vi "Local Trajectory Loading.vi"(6 "PID Cluster":T4={"L1 to L4 PID Cluster"={"L1 PID Gains"={"Kp"=0.005, "Kd"=0.5, "Ki"=0.0005}, "L2 PID Gains"={"Kp"=0.01, "Kd"=1.0, "Ki"=0.005}, "L3 PID Gains"={"Kp"=0.05, "Kd"=1.0, "Ki"=0.0005}, "L4 PID Gains"={"Kp"=0.1, "Kd"=0.1, "Ki"=0.0005}}, "Stage PID Cluster"={"Stage Z PID"={"Kp"=0.0005, "Kd"=0.001, "Ki"=0.0}, "Stage Y PID"={"Kp"=0.0003, "Kd"=0.01, "Ki"=0.0}, "Stage X PID"={"Kp"=0.0003, "Kd"=0.01, "Ki"=0.0}}, "OCT Z PID Gains"={"Kp"=0.0003, "Kd"=0.0001, "Ki"=0.01}}, 8 "error in":errorcluster, 9 "Offset Home 2 RCM":dbl[](array[numeric])=[0.0, 0.0, 0.0, 0.0], 10 "Prev Posit Cluster":T3={"Prev L1 to L4 Posit"=[-0.5319, -0.035669172703475985, -2.0566170657346783, 0.9099264705882353], "Prev Stage Posit"=[6.002553885707208, 5.996566124542428, 5.995469940427586], "Prev OCT Z Posit"=-0.0}, 11 "FPGA VI Reference In":refnum<k20>) -> (1 "Trajectory Cluster":T1, 2 "Last Posit Cluster":T2={"Last L1 to L4 Posit"=[0.0, 0.0, 0.0, 0.0], "Last Stage Posit"=[6.0, 6.0, 6.0], "Last OCT Z Posit"=0.0}, 3 "FPGA VI Reference Out":refnum<k20>, 4 "error out":errorcluster, 5 "First Trk Pt":dbl[](array[numeric]))   [LabVIEW 2016]
uses:
  <vilib>/Platform/TimedLoop/XDataNode/timing_clust.ctl
  <vilib>/Platform/TimedLoop/XDataNode/nitl_modes.ctl
  <vilib>/Platform/TimedLoop/XDataNode/wakeup.ctl
  Global Variables.vi
  <vilib>/platform/TimedLoop/XDataNode/XDataNode.xnode
  <vilib>/Platform/TimedLoop/XDataNode/XDNodeRunTimeDep.lvlib
panel:
  out "In Servo Loop":bool
  out "Loading Finished":bool
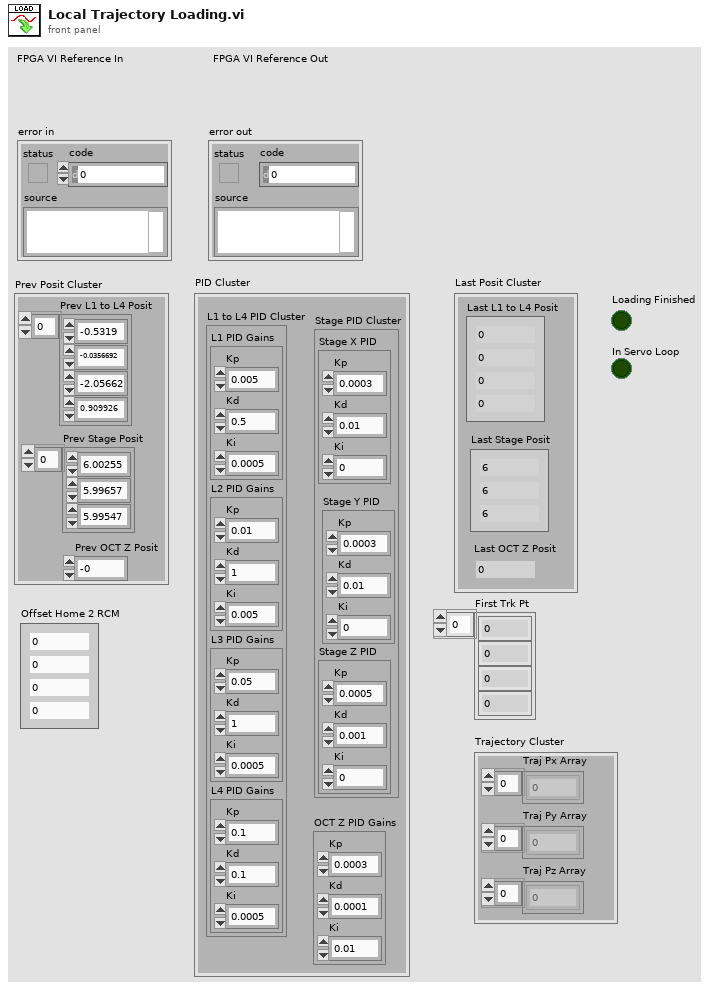
[diagram p1: front panel]
types:
  T1 = cluster{"Traj Px Array":dbl[], "Traj Py Array":dbl[], "Traj Pz Array":dbl[]}
  T2 = cluster{"Last L1 to L4 Posit":dbl[], "Last Stage Posit":dbl[], "Last OCT Z Posit":dbl}
  T3 = cluster{"Prev L1 to L4 Posit":dbl[], "Prev Stage Posit":dbl[], "Prev OCT Z Posit":dbl}
  T4 = cluster{"L1 to L4 PID Cluster":cluster{"L1 PID Gains":cluster{"Kp":dbl, "Kd":dbl, "Ki":dbl}, "L2 PID Gains":cluster{"Kp":dbl, "Kd":dbl, "Ki":dbl}, "L3 PID Gains":cluster{"Kp":dbl, "Kd":dbl, "Ki":dbl}, "L4 PID Gains":cluster{"Kp":dbl, "Kd":dbl, "Ki":dbl}}, "Stage PID Cluster":cluster{"Stage Z PID":cluster{"Kp":dbl, "Kd":dbl, "Ki":dbl}, "Stage Y PID":cluster{"Kp":dbl, "Kd":dbl, "Ki":dbl}, "Stage X PID":cluster{"Kp":dbl, "Kd":dbl, "Ki":dbl}}, "OCT Z PID Gains":cluster{"Kp":dbl, "Kd":dbl, "Ki":dbl}}
  T5 = typedef "XDNodeRunTimeDep.lvlib/timing_clust.ctl" = cluster{"Expected End [f-1]":u64, "Actual End [f-1]":u64, "Finished Late? [f-1]":bool, "Expected End [i-1]":u64, "Actual End [i-1]":u64, "Finished Late? [i-1]":bool, "Expected Start [i]":u64, "Actual Start [i]":u64, "Expected Start [f]":u64, "Actual Start [f]":u64, "Source Name":string, "Structure Name":string, "Period":i64, "Deadline":i64, "Offset":i64, "Start":i64, "Priority":i32, "Timeout":i32, "Mode":T6, "Wakeup Reason":T7, "Error":errorcluster, "Source Type":string, "Secondary Source Type":string, "Global End Time":u64, "Global Start Time":u64, "Frame Duration":u64, "Iteration Duration":u64, "Assigned CPU":i32, "I/O Scan Engine Mode":u32}
  T6 = typedef "XDNodeRunTimeDep.lvlib/nitl_modes.ctl" = enum32{"No Change", "Process missed periods, maintain original phase", "Discard missed periods, maintain original phase", "Process missed periods, ignore original phase", "Discard missed periods, ignore original phase"}
  T7 = typedef "XDNodeRunTimeDep.lvlib/wakeup.ctl" = enum32{"Normal", "Aborted", "Asynchronous wakeup", "Timing source error", "Timed loop error", "Timeout"}
  T8 = cluster{"L1 PID Gains":cluster{"Kp":dbl, "Kd":dbl, "Ki":dbl}, "L2 PID Gains":cluster{"Kp":dbl, "Kd":dbl, "Ki":dbl}, "L3 PID Gains":cluster{"Kp":dbl, "Kd":dbl, "Ki":dbl}, "L4 PID Gains":cluster{"Kp":dbl, "Kd":dbl, "Ki":dbl}}
  T9 = cluster{"Stage Z PID":cluster{"Kp":dbl, "Kd":dbl, "Ki":dbl}, "Stage Y PID":cluster{"Kp":dbl, "Kd":dbl, "Ki":dbl}, "Stage X PID":cluster{"Kp":dbl, "Kd":dbl, "Ki":dbl}}
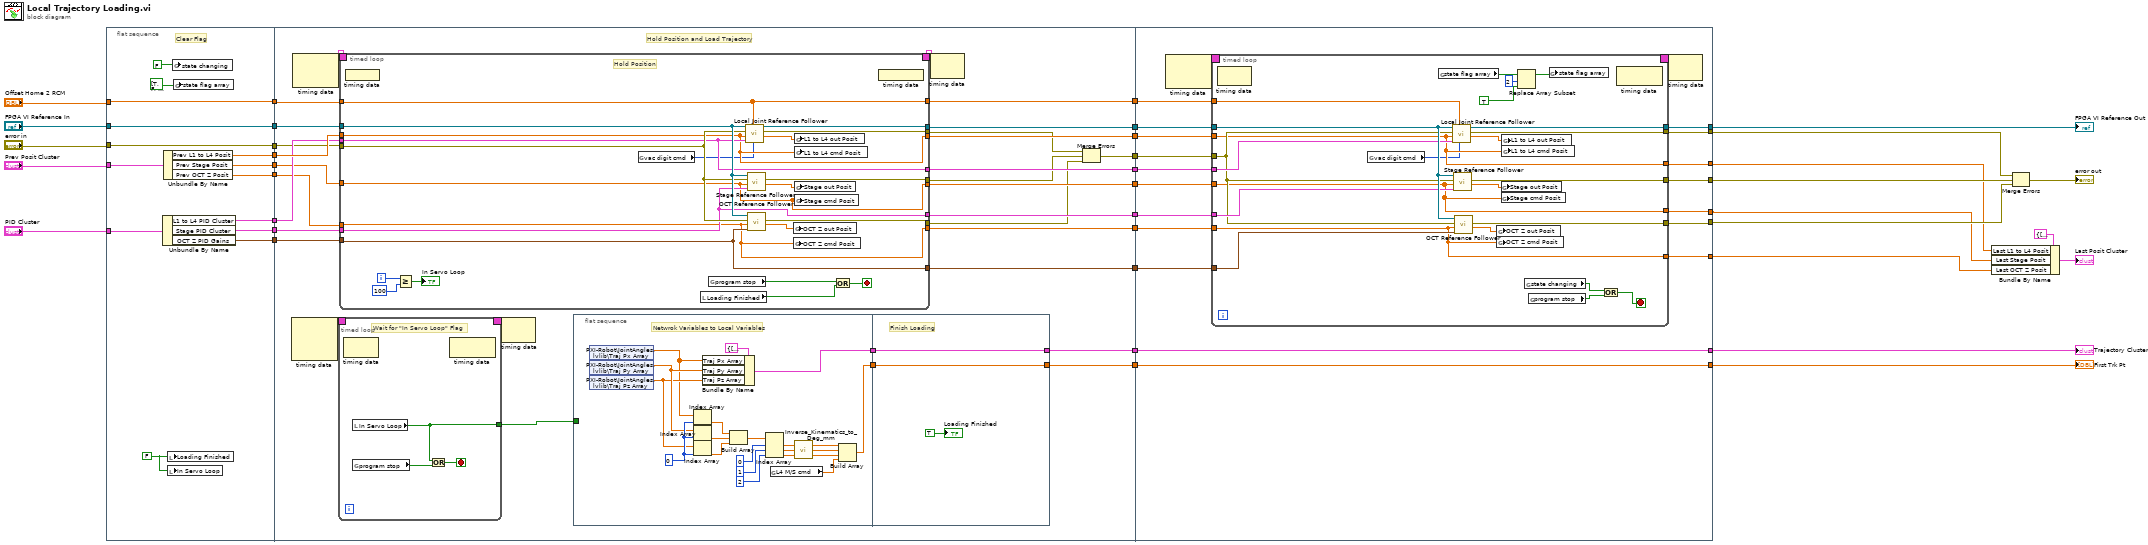
[diagram p0: block diagram]
diagram:
  n1 = flat-sequence {
    tunnel: [w49] -> w37
    tunnel: "FPGA VI Reference In" -> [w49]
    tunnel: [w48] -> w35
    tunnel: "error in" -> [w48]
    tunnel: "Prev Posit Cluster" -> [w47]
    tunnel: "PID Cluster" -> [w46]
    tunnel: [w45] -> w33
    tunnel: [w44] -> w32
    tunnel: "Offset Home 2 RCM" -> [w43]
    tunnel: [w43] -> w30
    tunnel: [w42] -> w27
    tunnel: [w41] -> w26
    tunnel: [w40] -> w25
    tunnel: [w39] -> w24
    tunnel: w37 -> [w67]
    tunnel: w35 -> [w62]
    tunnel: w33 -> [w64]
    tunnel: w32 -> [w63]
    tunnel: w30 -> [w68]
    tunnel: w27 -> [w66]
    tunnel: w26 -> [w61]
    tunnel: w25 -> [w60]
    tunnel: w24 -> [w65]
    tunnel: [w81] -> w12
    tunnel: [w80] -> w11
    tunnel: [w79] -> w10
    tunnel: [w78] -> w9
    tunnel: [w77] -> w8
    tunnel: [w76] -> w7
    tunnel: [w75] -> w6
    tunnel: [w74] -> w5
    tunnel: [w56] -> w4
    tunnel: [w55] -> w3
    tunnel: [w54] -> w2
    tunnel: w12 -> [w157]
    tunnel: [w156] -> w22
    tunnel: [w155] -> w21
    tunnel: [w154] -> w20
    tunnel: w11 -> [w153]
    tunnel: w10 -> [w152]
    tunnel: w9 -> [w151]
    tunnel: w8 -> [w150]
    tunnel: w7 -> [w149]
    tunnel: w6 -> [w148]
    tunnel: w5 -> [w147]
    tunnel: [w146] -> w18
    tunnel: [w145] -> w17
    tunnel: [w144] -> w16
    tunnel: [w143] -> w14
    tunnel: [w140] -> w13
    tunnel: w4 -> [w142]
    tunnel: w3 -> [w140]
    tunnel: [w141] -> w1
    tunnel: w2 -> [w141]
    frame #0 {
      w38 = FALSE ("Loading Finished")
      # "Clear Flag"
      n2 = Unbundle By Name(w46) -> ("L1 to L4 PID Cluster"=w44:T8, "Stage PID Cluster"=w45:T9, "OCT Z PID Gains"=w39:cluster{"Kp":dbl, "Kd":dbl, "Ki":dbl})
      n3 = Unbundle By Name(w47) -> ("Prev L1 to L4 Posit"=w42:dbl[], "Prev Stage Posit"=w41:dbl[], "Prev OCT Z Posit"=w40:dbl)
      n4 = local write "Loading Finished"(w38) -> ()
      n5 = local write "In Servo Loop"(w38) -> ()
      n6 = global write "Global Variables.vi" "state changing"(FALSE ("state changing")) -> ()
      n7 = global write "Global Variables.vi" "state flag array"(bool[] [TRUE, FALSE, FALSE, FALSE, FALSE, FALSE, FALSE, FALSE, FALSE] ("state flag array")) -> ()
    }
    frame #1 {
      # "Hold Position and Load Trajectory"
      n8 = node-c288() -> (w71:T5)  [unwired: 3 in]
      n9 = node-c288() -> (w73:T5)  [unwired: 2 in]
      n10 = timed-loop {
        timing: w71 -> [_]
        timing-out: [_] -> w70
        tunnel: [w83] -> w69
        stop <- w84 stop-if-true
        # "Wait for \"In Servo Loop\" Flag"
        n11 = node-c288() -> ()  [unwired: 1 in, 1 out]
        n12 = local read "In Servo Loop"() -> (w83:bool)
        n13 = global read "Global Variables.vi" "program stop"() -> (w82:bool)
        n14 = Or(x=w83, y=w82) -> (x .or. y?=w84:bool)
        n15 = node-c288() -> ()  [unwired: 1 in, 1 out]
      }
      n16 = timed-loop {
        timing: w73 -> [_]
        timing-out: [_] -> w72
        tunnel: w66 -> [w116]
        tunnel: w61 -> [w115]
        tunnel: w64 -> [w120]
        tunnel: w63 -> [w121]
        tunnel: w62 -> [w131]
        tunnel: w67 -> [w132]
        tunnel: w68 -> [w127]
        tunnel: w60 -> [w114]
        tunnel: w65 -> [w122]
        tunnel: [w116] -> w79
        tunnel: [w115] -> w78
        tunnel: [w114] -> w77
        tunnel: [w127] -> w80
        tunnel: [w126] -> w81
        tunnel: [w125] -> w59
        tunnel: [w124] -> w58
        tunnel: [w123] -> w57
        tunnel: [w122] -> w76
        tunnel: [w121] -> w75
        tunnel: [w120] -> w74
        i -> [w119]
        stop <- w135 stop-if-true
        # "Hold Position"
        n17 = node-c288 ("Output Node")() -> ()  [unwired: 1 in]
        n18 = Greater Or Equal?(x=w119, y=100) -> (x >= y?=→"In Servo Loop":bool)
        n19 = global read "Global Variables.vi" "vac digit cmd"() -> (w113:i8)
        n20 = local read "Loading Finished"() -> (w134:bool)
        n21 = global read "Global Variables.vi" "program stop"() -> (w133:bool)
        n22 = call "Local Joint Reference Follower.vi"("Digital Cmd [0-78]"=w113, "Offset Home2RCM [deg/mm]"=w127, "PID Ctrl Cluster"=w121, "Ref Array [deg/mm]"=w116, "error in"=w131, "FPGA VI Reference In"=w132) -> ("Output Posit Array [deg/mm]"=w130:dbl[], "error out"=w125:errorcluster, "FPGA VI Reference Out"=w126:refnum<k20>)  [unwired: 3 in]
        n23 = call "Stage Reference Follower.vi"("Stage PID Cluster"=w120, "Stage cmd Posit [mm]"=w115, "error in"=w131, "FPGA VI Reference In"=w132) -> ("Stage out Posit [mm]"=w129:dbl[], "error out"=w124:errorcluster)  [unwired: 5 in, 1 out]
        n24 = call "OCT Reference Follower.vi"("OCT Z PID Gains"=w122, "OCT  Z cmd Posit [mm]"=w114, "error in"=w131, "FPGA VI Reference In"=w132) -> ("OCT  Z out Posit [mm]"=w128:dbl, "error out"=w123:errorcluster)  [unwired: 5 in, 1 out]
        n25 = global write "Global Variables.vi" "OCT Z out Posit"(w128) -> ()
        n26 = global write "Global Variables.vi" "OCT Z cmd Posit"(w114) -> ()
        n27 = global write "Global Variables.vi" "L1 to L4 out Posit"(w130) -> ()
        n28 = global write "Global Variables.vi" "L1 to L4 cmd Posit"(w116) -> ()
        n29 = global write "Global Variables.vi" "Stage out Posit"(w129) -> ()
        n30 = global write "Global Variables.vi" "Stage cmd Posit"(w115) -> ()
        n31 = Or(x=w133, y=w134) -> (x .or. y?=w135:bool)
        n32 = node-c288() -> ()  [unwired: 1 out]
      }
      n33 = node-c288(w70) -> ()  [unwired: 1 out]
      n34 = flat-sequence {
        tunnel: [w108] -> w53
        tunnel: w69 -> [_]
        tunnel: [w91] -> w52
        tunnel: w53 -> [w111]
        tunnel: [w111] -> w55
        tunnel: [w110] -> w54
        tunnel: w52 -> [w110]
        frame #0 {
          w106 = 0 ("index")
          # "Netwrok Variables to Local Variables"
          n35 = shared-variable "PXI-Robot\\JointAngles.lvlib\\Traj Px Array"() -> (w89:dbl[])  [unwired: 1 in, 1 out]
          n36 = shared-variable "PXI-Robot\\JointAngles.lvlib\\Traj Py Array"() -> (w93:dbl[])  [unwired: 1 in, 1 out]
          n37 = shared-variable "PXI-Robot\\JointAngles.lvlib\\Traj Pz Array"() -> (w92:dbl[])  [unwired: 1 in, 1 out]
          n38 = Index Array(array=w89, index=w106) -> (element=w94:dbl)
          n39 = Index Array(array=w93, index=w106) -> (element=w95:dbl)
          n40 = Index Array(array=w92, index=w106) -> (element=w96:dbl)
          n41 = Bundle By Name(cluster=T1 {"Traj Px Array"=[], "Traj Py Array"=[], "Traj Pz Array"=[]} ("Trajectory Cluster"), "Traj Px Array"=w89, "Traj Py Array"=w93, "Traj Pz Array"=w92) -> (w108:T1)
          n42 = Build Array(w94, w95, w96) -> (w107:dbl[])
          n43 = Index Array(array=w107, index #1=0 ("index"), index #2=1 ("index"), index #3=2 ("index")) -> (element #1=w101:dbl, element #2=w103:dbl, element #3=w102:dbl)
          n44 = global read "Global Variables.vi" "L4 M/S cmd"() -> (w90:dbl)
          n45 = call "Inverse_Kinematics_to_Deg_mm.vi"("pz"=w102, "py"=w103, "px"=w101) -> ("L3 [mm]"=w98:dbl, "L2 [deg]"=w99:dbl, "L1 [deg]"=w100:dbl)
          n46 = Build Array(w100, w99, w98, w90) -> (w91:dbl[])
        }
        frame #1 {
          # "Finish Loading"
          "Loading Finished" <- TRUE ("Loading Finished")
        }
      }
      n47 = node-c288(w72) -> ()  [unwired: 1 out]
      n48 = Merge Errors(w59, w58, w57) -> (w56:errorcluster)
    }
    frame #2 {
      n49 = node-c288() -> (w159:T5)  [unwired: 2 in]
      n50 = timed-loop {
        timing: w159 -> [_]
        timing-out: [_] -> w158
        tunnel: w157 -> [w176]
        tunnel: [w175] -> w155
        tunnel: [w174] -> w156
        tunnel: [w173] -> w154
        tunnel: w153 -> [w172]
        tunnel: w152 -> [w163]
        tunnel: w151 -> [w162]
        tunnel: w150 -> [w161]
        tunnel: w149 -> [w171]
        tunnel: w148 -> [w170]
        tunnel: w147 -> [w169]
        tunnel: [w163] -> w146
        tunnel: [w162] -> w145
        tunnel: [w161] -> w144
        tunnel: [w165] -> w143
        tunnel: w142 -> [w164]
        stop <- w183 stop-if-true
        n51 = node-c288() -> ()  [unwired: 1 in, 1 out]
        n52 = global read "Global Variables.vi" "vac digit cmd"() -> (w160:i8)
        n53 = global read "Global Variables.vi" "state flag array"() -> (w180:bool[])
        n54 = call "Local Joint Reference Follower.vi"("Digital Cmd [0-78]"=w160, "Offset Home2RCM [deg/mm]"=w172, "PID Ctrl Cluster"=w170, "Ref Array [deg/mm]"=w163, "error in"=w164, "FPGA VI Reference In"=w176) -> ("Output Posit Array [deg/mm]"=w168:dbl[], "error out"=w175:errorcluster, "FPGA VI Reference Out"=w165:refnum<k20>)  [unwired: 3 in]
        n55 = call "Stage Reference Follower.vi"("Stage PID Cluster"=w169, "Stage cmd Posit [mm]"=w162, "error in"=w164, "FPGA VI Reference In"=w176) -> ("Stage out Posit [mm]"=w167:dbl[], "error out"=w174:errorcluster)  [unwired: 5 in, 1 out]
        n56 = call "OCT Reference Follower.vi"("OCT Z PID Gains"=w171, "OCT  Z cmd Posit [mm]"=w161, "error in"=w164, "FPGA VI Reference In"=w176) -> ("OCT  Z out Posit [mm]"=w166:dbl, "error out"=w173:errorcluster)  [unwired: 5 in, 1 out]
        n57 = global write "Global Variables.vi" "OCT Z out Posit"(w166) -> ()
        n58 = global write "Global Variables.vi" "OCT Z cmd Posit"(w161) -> ()
        n59 = global write "Global Variables.vi" "Stage out Posit"(w167) -> ()
        n60 = global write "Global Variables.vi" "Stage cmd Posit"(w162) -> ()
        n61 = global write "Global Variables.vi" "L1 to L4 out Posit"(w168) -> ()
        n62 = global write "Global Variables.vi" "L1 to L4 cmd Posit"(w163) -> ()
        n63 = Replace Array Subset(array=w180, new element=TRUE ("new element/subarray"), index=2) -> (w179:bool[])
        n64 = global read "Global Variables.vi" "state changing"() -> (w182:bool)
        n65 = global read "Global Variables.vi" "program stop"() -> (w181:bool)
        n66 = global write "Global Variables.vi" "state flag array"(w179) -> ()
        n67 = Or(x=w182, y=w181) -> (x .or. y?=w183:bool)
        n68 = node-c288() -> ()  [unwired: 1 in, 1 out]
      }
      n69 = node-c288(w158) -> ()  [unwired: 1 out]
    }
  }
  n70 = Bundle By Name(cluster=T2 {"Last L1 to L4 Posit"=[0.0, 0.0, 0.0, 0.0], "Last Stage Posit"=[6.0, 6.0, 6.0], "Last OCT Z Posit"=0.0} ("Last Posit Cluster 2"), "Last L1 to L4 Posit"=w18, "Last Stage Posit"=w17, "Last OCT Z Posit"=w16) -> (→"Last Posit Cluster":T2)
  n71 = Merge Errors(w21, w22, w20) -> (→"error out":errorcluster)
  "FPGA VI Reference Out" <- w14
  "First Trk Pt" <- w1
  "Trajectory Cluster" <- w13
